vi "Enlarge_Old_Array.vi"(8 "new input array":dbl[][](array[numeric]), 11 "old input array (IN)":dbl[][](array[numeric])) -> (3 "old input array (OUT)":dbl[][](array[numeric]))   [LabVIEW 2013]
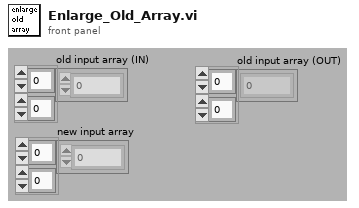
[diagram p1: front panel]
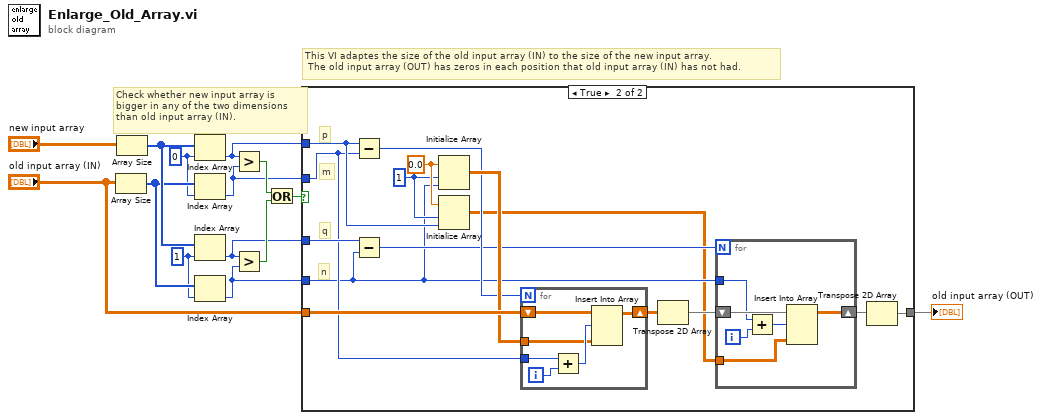
[diagram p0: block diagram]
diagram:
  w11 = 1 ("index")
  w12 = 0 ("index")
  # "Check whether new input array is\nbigger in any of the two dimensions\nthan old input array (IN)."
  # "This VI adaptes the size of the old input array (IN) to the size of the new input array.\n The old input array (OUT) has zeros in each position that old input array (IN) has not had."
  n1 = Array Size(array="old input array (IN)") -> (size(s)=w13:i32[])
  n2 = Array Size(array="new input array") -> (size(s)=w14:i32[])
  n3 = Index Array(array=w14, index=w12) -> (element=w7:i32)
  n4 = Index Array(array=w13, index=w12) -> (element=w6:i32)
  n5 = Index Array(array=w14, index=w11) -> (element=w5:i32)
  n6 = Index Array(array=w13, index=w11) -> (element=w4:i32)
  n7 = Greater?(x=w7, y=w6) -> (0:w10:bool)
  n8 = Greater?(x=w5, y=w4) -> (0:w9:bool)
  n9 = Or(x=w10, y=w9) -> (x .or. y?=w8:bool)
  n10 = case shown="True" w8 {
    tunnel: "old input array (IN)" -> [w15 w27]
    tunnel: [w15 w17] -> w1
    tunnel: w7 -> [_ w21]
    tunnel: w6 -> [_ w20]
    tunnel: w5 -> [_ w29]
    tunnel: w4 -> [_ w19]
    frame False {
    }
    frame True {
      w28 = 1 ("dimension size")
      w30 = 0.0 ("element")
      # "n"
      # "q"
      # "m"
      # "p"
      n11 = Subtract(x=w21, y=w20) -> (x-y=w25:i32)
      n12 = Subtract(x=w29, y=w19) -> (x-y=w22:i32)
      n13 = Initialize Array(w30, w28, w19) -> (w26:dbl[][])
      n14 = Initialize Array(w30, w28, w21) -> (w16:dbl[][])
      n15 = for {
        N: w25 -> [_]
        shift-right: [w41] -> w24
        shift-left: w27 -> [w42]
        tunnel: w20 -> [w39]
        tunnel: w26 -> [w37]
        i -> [w40]
        n16 = Add(x=w39, y=w40) -> (x+y=w38:i32)
        n17 = Insert Into Array(array=w42, index (row)=w38, new element=w37) -> (w41:dbl[][])  [unwired: 1 in]
      }
      n18 = Transpose 2D Array(2D array=w24) -> (transposed array=w23:dbl[][])
      n19 = for {
        N: w22 -> [_]
        shift-right: [w32] -> w18
        shift-left: w23 -> [w36]
        tunnel: w19 -> [w34]
        tunnel: w16 -> [w31]
        i -> [w35]
        n20 = Add(x=w34, y=w35) -> (x+y=w33:i32)
        n21 = Insert Into Array(array=w36, index (row)=w33, new element=w31) -> (w32:dbl[][])  [unwired: 1 in]
      }
      n22 = Transpose 2D Array(2D array=w18) -> (transposed array=w17:dbl[][])
    }
  }
  "old input array (OUT)" <- w1
